vi "Write Motor Command.vi"(8 "error in (no error)":errorcluster, 9 "Motor Command":i16, 10 "Motor":T1, 11 "MCB Command in":refnum<class "MCB Command.lvclass">) -> (0 "error out":errorcluster, 3 "MCB Command out":refnum<class "MCB Command.lvclass">)   [LabVIEW 2015, in "RDS Child Messages.lvlib" / "MCB Command.lvclass"]
uses:
  MCB Command.lvclass
  MCB Channel.ctl
  MCB Command.lvclass/MCB Command.ctl
  RDS Child Messages.lvlib
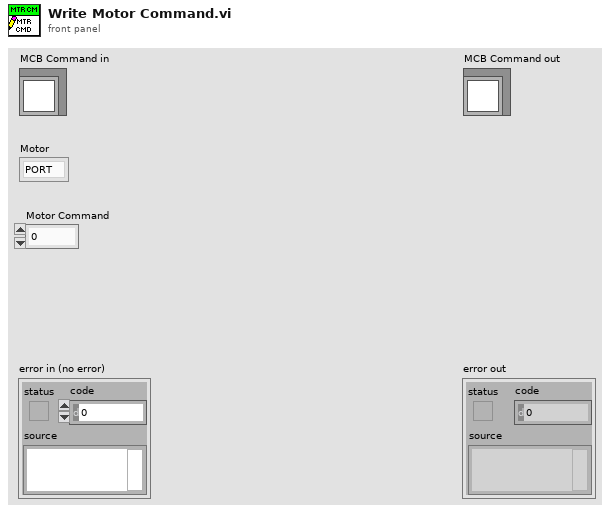
[diagram p1: front panel]
types:
  T1 = typedef "RDS Child Messages.lvlib/MCB Channel.ctl" = enum16{"PORT", "STBD"}
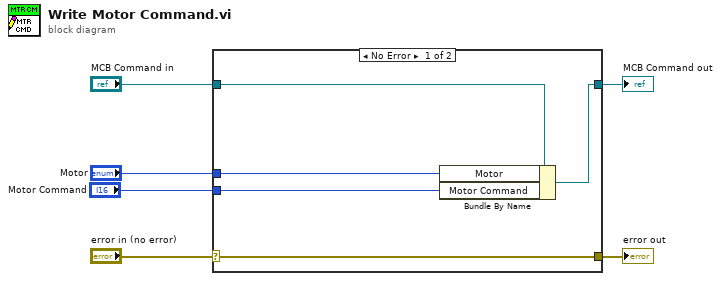
[diagram p0: block diagram]
diagram:
  n1 = case shown="No Error" "error in (no error)" {
    selector: "error in (no error)" -> [w11 w12]
    tunnel: [w11 w12] -> w5
    tunnel: [w9 w13] -> w3
    tunnel: "MCB Command in" -> [w10 w13]
    tunnel: "Motor" -> [w8 _]
    tunnel: "Motor Command" -> [w7 _]
    frame No Error {
      n2 = Bundle By Name(cluster=w10, "Motor"=w8, "Motor Command"=w7) -> (w9:refnum<class "MCB Command.lvclass">)
    }
    frame Error {
    }
  }
  "error out" <- w5
  "MCB Command out" <- w3
